vi "Demo.vi"() -> ()   [LabVIEW 2020, in "Process Generation.lvlib" / "Tag Tree Helper.lvclass"]
uses:
  Tag Tree Helper.lvclass
panel:
  out "Selected Tags":string[](array[string])
  in  "Tree":string[](tree)
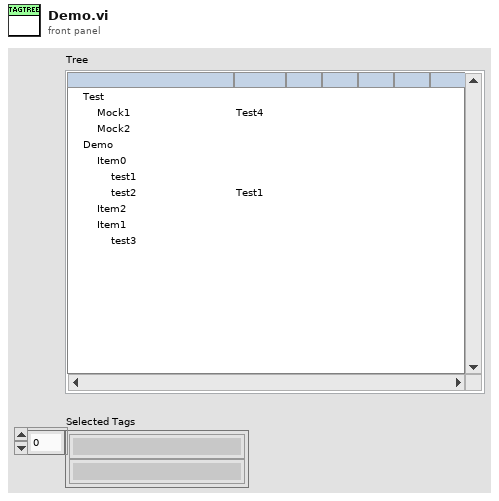
[diagram p1: front panel]
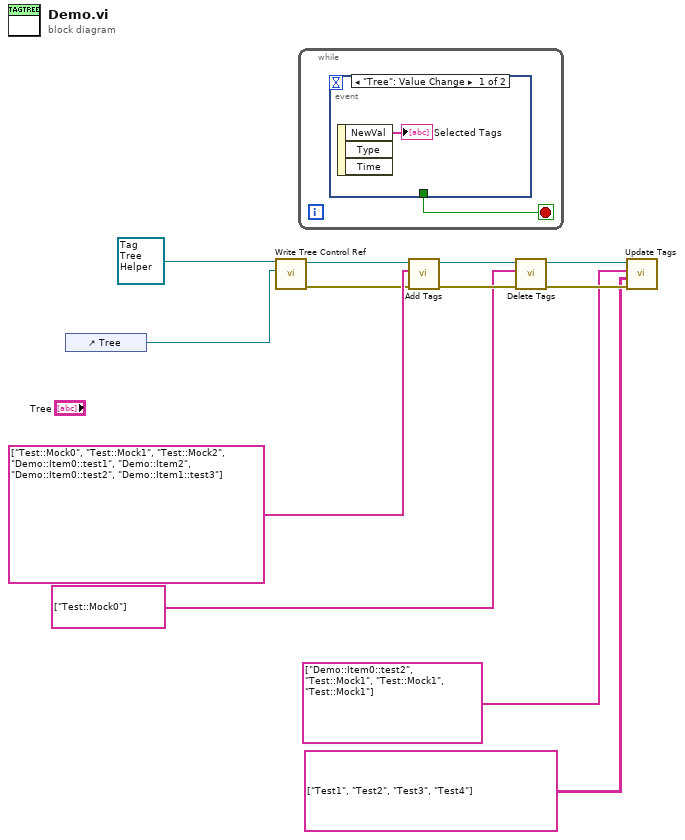
[diagram p0: block diagram]
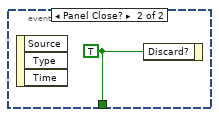
[diagram p2: hidden frame]
diagram:
  n1 = control-ref of="Tree"() -> (w11:refnum<vi>)
  n2 = call "Write Tree Control Ref.vi"("Tag Tree Reference"=w11, "Tag Tree Helper In"=refnum<class "Tag Tree Helper.lvclass"> refnum ("Support Utilities.lvlib:Tag Tree.lvclass")) -> ("error out"=w8:errorcluster, "Tag Tree Helper Out"=w10:refnum<class "Tag Tree Helper.lvclass">)  [unwired: 8 in]
  n3 = while {
    stop <- w13 stop-if-true
    n4 = event shown="[0] \"Tree\": Value Change" {
      selector: _ -> [_ _]
      dyn-events: _ -> [_ _]
      timeout: _ -> [_ _]
      tunnel: [_ w15] -> w13
      event "Tree": Value Change {
        n5 = event-data() -> ("NewVal"=→"Selected Tags":string[])  [unwired: 1 in, 2 out]
      }
      event Panel Close? {
        w15 = TRUE ("Discard?")
        n6 = event-data() -> ()  [unwired: 1 in, 3 out]
        n7 = event-data ("Event Filter Node")("Discard?"=w15) -> ()  [unwired: 1 in, 1 out]
      }
    }
  }
  n8 = call "Add Tags.vi"("error in (no error)"=w8, "Tag"=string[] ["Test::Mock0", "Test::Mock1", "Test::Mock2", "Demo::Item0::test1", "Demo::Item2", "Demo::Item0::test2", "Demo::Item1::test3"], "Tag Tree Helper In"=w10) -> ("error out"=w6:errorcluster, "Tag Tree Helper Out"=w7:refnum<class "Tag Tree Helper.lvclass">)  [unwired: 7 in]
  n9 = call "Delete Tags.vi"("error in (no error)"=w6, "Tag"=string[] ["Test::Mock0"], "Tag Tree Helper In"=w7) -> ("error out"=w4:errorcluster, "Tag Tree Helper Out"=w3:refnum<class "Tag Tree Helper.lvclass">)  [unwired: 7 in]
  n10 = call "Update Tags.vi"("error in (no error)"=w4, "Child Text"=string[][] [["Test1"], ["Test2"], ["Test3"], ["Test4"]], "Tag"=string[] ["Demo::Item0::test2", "Test::Mock1", "Test::Mock1", "Test::Mock1"], "Tag Tree Helper In"=w3) -> ()  [unwired: 6 in, 2 out]
